vi "RecursiveClusterValueSet.vi"(0 "Controls[] In":refnum<vi>[](array[refnum]), 5 "Array":string[](array[string]), 7 "Control Value":variant, 11 "error in (no error)":errorcluster) -> (4 "Controls[] Out":refnum<vi>[](array[refnum]), 15 "error out":errorcluster)   [LabVIEW 2016]
uses:
  <vilib>/ErrorRing/Error Ring.xnode
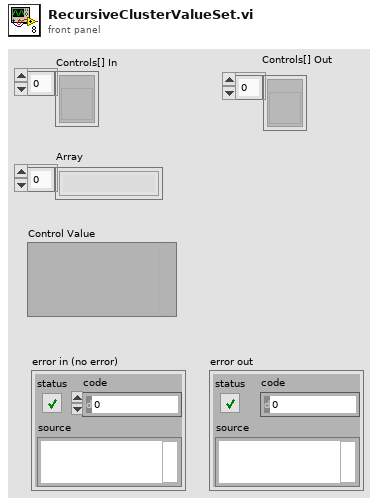
[diagram p1: front panel]
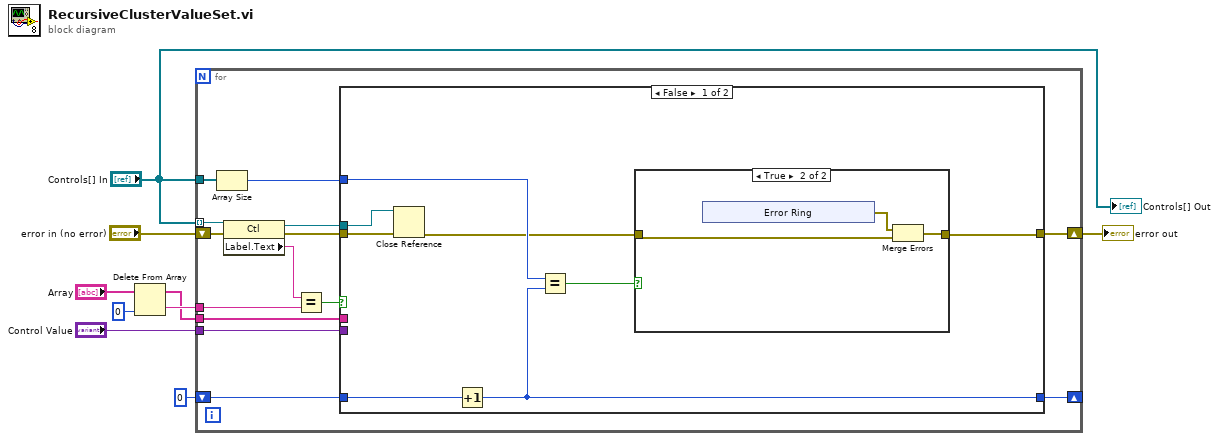
[diagram p0: block diagram]
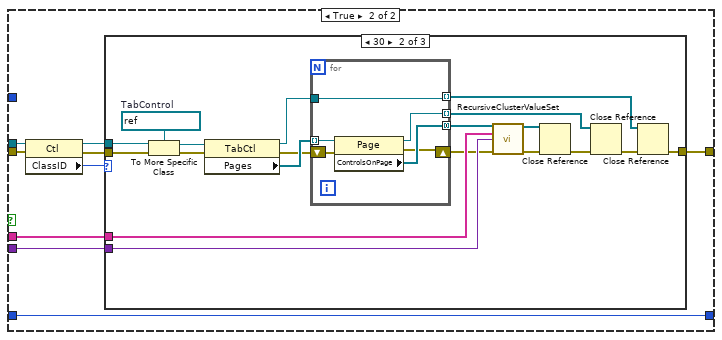
[diagram p3: hidden frame]
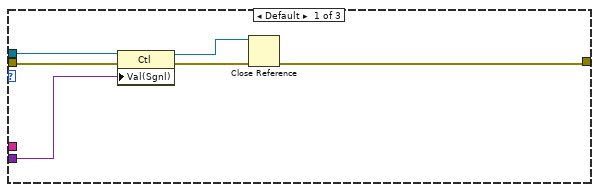
[diagram p4: hidden frame]
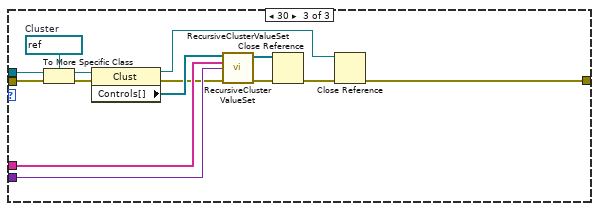
[diagram p5: hidden frame]
diagram:
  n1 = Delete From Array(array="Array", index=0) -> (deleted portion=w7:string, array with subset deleted=w6:string[])  [unwired: 1 in]
  n2 = for {
    tunnel: "Controls[] In" -> [w23] mode=indexing
    tunnel: w7 -> [w20]
    tunnel: w6 -> [w18]
    tunnel: "Control Value" -> [w17]
    shift-right: [w14] -> w2
    shift-left: "error in (no error)" -> [w16]
    tunnel: "Controls[] In" -> [w13]
    shift-right: [w10] -> _
    shift-left: 0 -> [w11]
    n3 = Array Size(array=w13) -> (size(s)=w12:i32)
    n4 = property class="Ctl"(reference=w23, error in=w16) -> (reference out=w19:refnum<vi>, error out=w15:errorcluster, "Label.Text"=w21:string)
    n5 = Equal?(x=w21, y=w20) -> (x = y?=w22:bool)
    n6 = case shown="False" w22 {
      tunnel: w19 -> [w31 w45]
      tunnel: w18 -> [_ w43]
      tunnel: w17 -> [_ w42]
      tunnel: w15 -> [w30 w41]
      tunnel: [w25 w39] -> w14
      tunnel: w12 -> [w27 _]
      tunnel: w11 -> [w29 w38]
      tunnel: [w28 w38] -> w10
      frame False {
        n7 = Close Reference(reference=w31, error in (no error)=w30) -> (error out=w24:errorcluster)
        n8 = Increment(x=w29) -> (x+1=w28:i32)
        n9 = Equal?(x=w27, y=w28) -> (x = y?=w26:bool)
        n10 = case shown="True" w26 {
          tunnel: [w32 w35] -> w25
          tunnel: w24 -> [w32 w33]
          frame False {
          }
          frame True {
            n11 = xnode "Error Ring"() -> ("error out"=w34:errorcluster)
            n12 = Merge Errors(w34, w33) -> (w35:errorcluster)
          }
        }
      }
      frame True {
        n13 = property class="Ctl"(reference=w45, error in=w41) -> (reference out=w37:refnum<vi>, error out=w40:errorcluster, "ClassID"=w44:u32)
        n14 = case shown="30" w44 {
          tunnel: w37 -> [w51 w67 w90]
          tunnel: w43 -> [_ w63 w84]
          tunnel: w42 -> [w50 w62 w83]
          tunnel: w40 -> [w49 w65 w86]
          tunnel: [w47 w55 w78] -> w39
          frame Default {
            n15 = property class="Ctl"(reference=w51, error in=w49, "Val(Sgnl)"=w50) -> (reference out=w46:refnum<vi>, error out=w48:errorcluster)
            n16 = Close Reference(reference=w46, error in (no error)=w48) -> (error out=w47:errorcluster)
          }
          frame 55 {
            w70 = refnum<vi> refnum  # TabControl
            n17 = To More Specific Class(target class=w70, reference=w67, error in=w65) -> (specific class reference=w69:refnum<vi>, error out=w68:errorcluster)
            n18 = property class="TabCtl"(reference=w69, error in=w68) -> (reference out=w59:refnum<vi>, error out=w60:errorcluster, "Pages"=w66:refnum<vi>[])
            n19 = for {
              tunnel: w66 -> [w76] mode=indexing
              tunnel: [w75] -> w64 mode=concatenating
              shift-right: [w73] -> w61
              shift-left: w60 -> [w74]
              tunnel: [w72] -> w53 mode=indexing
              tunnel: [w71] -> w52 mode=indexing
              tunnel: w59 -> [w71]
              n20 = property class="Page"(reference=w76, error in=w74) -> (reference out=w72:refnum<vi>, error out=w73:errorcluster, "ControlsOnPage"=w75:refnum<vi>[])
            }
            n21 = call "RecursiveClusterValueSet.vi"("Controls[] In"=w64, "Array"=w63, "Control Value"=w62, "error in (no error)"=w61) -> ("Controls[] Out"=w54:refnum<vi>[], "error out"=w56:errorcluster)  [unwired: 10 in]
            n22 = Close Reference(reference=w54, error in (no error)=w56) -> (error out=w58:errorcluster)
            n23 = Close Reference(reference=w53, error in (no error)=w58) -> (error out=w57:errorcluster)
            n24 = Close Reference(reference=w52, error in (no error)=w57) -> (error out=w55:errorcluster)
          }
          frame 30 {
            w89 = refnum<vi> refnum  # Cluster
            n25 = To More Specific Class(target class=w89, reference=w90, error in=w86) -> (specific class reference=w88:refnum<vi>, error out=w87:errorcluster)
            n26 = property class="Clust"(reference=w88, error in=w87) -> (reference out=w77:refnum<vi>, error out=w82:errorcluster, "Controls[]"=w85:refnum<vi>[])
            n27 = call "RecursiveClusterValueSet.vi"() -> ("Controls[] Out"=w80:refnum<vi>[], "error out"=w81:errorcluster)  [unwired: 14 in]
            n28 = call "RecursiveClusterValueSet.vi"("Controls[] In"=w85, "Array"=w84, "Control Value"=w83, "error in (no error)"=w82) -> ()  [unwired: 10 in, 2 out]
            n29 = Close Reference(reference=w80, error in (no error)=w81) -> (error out=w79:errorcluster)
            n30 = Close Reference(reference=w77, error in (no error)=w79) -> (error out=w78:errorcluster)
          }
        }
      }
    }
  }
  "error out" <- w2
  "Controls[] Out" <- "Controls[] In"
